vi "Host_FastOsziTest_ContAcq.vi"() -> ()   [LabVIEW 2012]
uses:
  <vilib>/FPGAPlugInAG/PXIe-7962R/niLvFpga_Open_PXIe-7962R.vi
  <vilib>/rvi/interface/common/dynamic/niFpgaDynamicAddResources.vi
  <vilib>/Utility/error.llb/Error Cluster From Error Code.vi
  <vilib>/rvi/errors/niLvFpgaAdjustHostInterfaceError.vi
  <vilib>/FPGAPlugInAG/Dynamic/niLvFpga_Close_Dynamic.vi
  <vilib>/rvi/interface/nirviOpenFPGA/nirviOpenFPGA.xnode
  FPGA Bitfiles/AnalogIntegratorFastOszi_NI5771_PXIe-7962R.lvbitx
  FPGA VIs/AnalogIntegratorFastOszi_NI5771.vi
  <vilib>/rvi/interface/nirviMethod/nirviMethod.xnode
  <vilib>/rvi/interface/nirviReadWriteControl/nirviReadWriteControl.xnode
  <vilib>/rvi/interface/nirviCloseFPGA/nirviCloseFPGA.xnode
  <vilib>/rvi/interface/Simulation/niFpgaSimulationCallBeginRW.vi
  NiFpgaLv.dll
  <vilib>/FPGAPlugInAG/Dynamic/niLvFpga_ReadFifo_Dynamic.vi
  <vilib>/rvi/errors/niLvFpgaMergeErrorWithErrorCode.vi
  <vilib>/FPGAPlugInAG/Dynamic/niLvFpga_ConfigureFifo_Dynamic.vi
panel:
  in  "Acquire continuously":bool=TRUE
  out "Configured?":bool
  out "ToHostCh1FIFO Overflow":bool
  out "InterloopFIFO Timeout":bool
  out "InterloopFIFO Overflow":bool
  in  "stop":bool
  out "Laser (Trigger In)":i16[](graph)
  in  "Samples to acquire":u32=10000
  out "IO Module\\AI Over Range":bool
  out "PMT (AI 0)":u8[](graph)
  # "Sampling at 1.5GHz => 0.66 ns sampling interval"
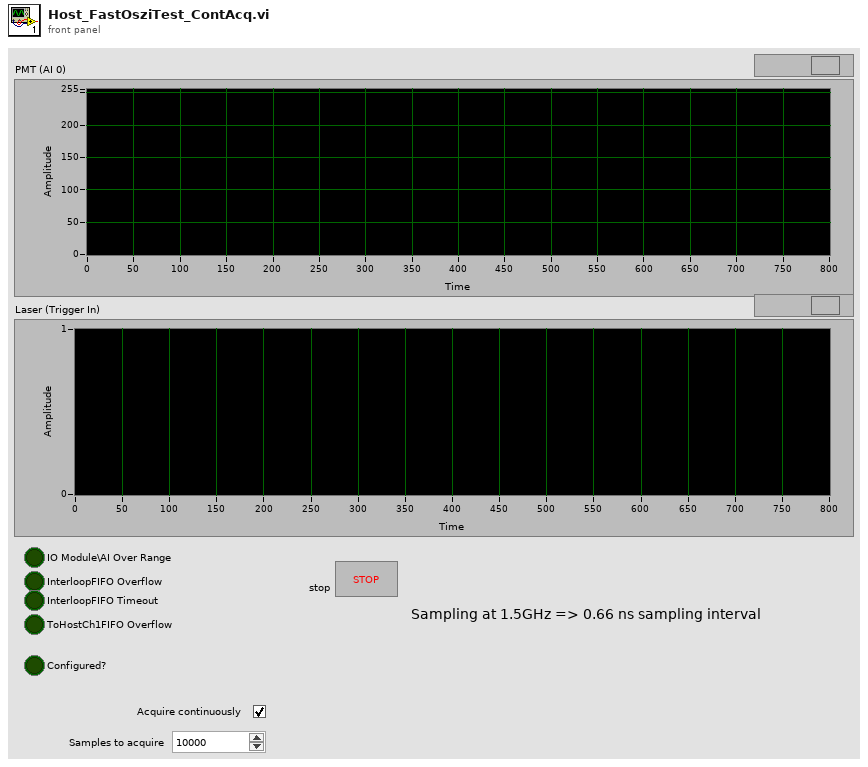
[diagram p1: front panel]
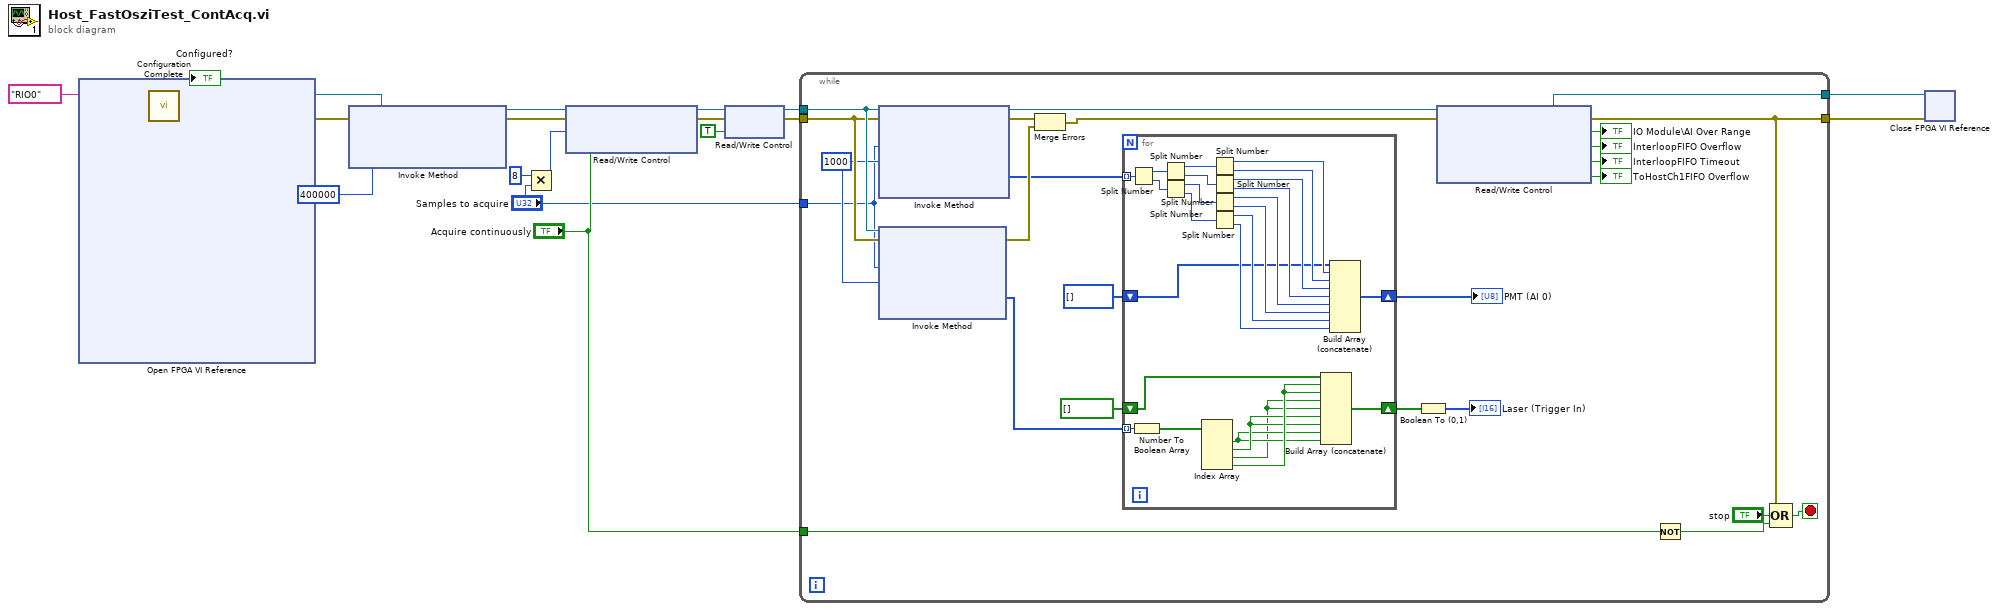
[diagram p0: block diagram]
diagram:
  n1 = xnode "Open FPGA VI Reference"("resource name"=tag "RIO0") -> ("FPGA VI Reference Out"=w15:refnum<k20>, "error out"=w19:errorcluster)  [unwired: 1 in]
  n2 = call "Configuration Complete.vi"("error in"=w19, "FPGA VI Reference In"=w15) -> ("error out"=w7:errorcluster, "Configured?"=→"Configured?":bool, "FPGA VI Reference Out"=w8:refnum<k20>)  [unwired: 7 in]
  n3 = xnode "Invoke Method"("FPGA VI Reference In"=w8, "error in"=w7, "Requested Depth"=u32 400000) -> ("FPGA VI Reference Out"=w5:refnum<k20>, "error out"=w6:errorcluster)  [unwired: 1 out]
  n4 = Multiply(x=u32 8, y="Samples to acquire") -> (x*y=w12:u32)
  n5 = xnode "Read/Write Control"("FPGA VI Reference In"=w5, "error in"=w6, "Samples to acquire"=w12, "Acquire continuously"="Acquire continuously") -> ("FPGA VI Reference Out"=w17:refnum<k20>, "error out"=w18:errorcluster)
  n6 = xnode "Read/Write Control"("FPGA VI Reference In"=w17, "error in"=w18, "Acquire"=TRUE) -> ("FPGA VI Reference Out"=w11:refnum<k20>, "error out"=w10:errorcluster)
  n7 = while {
    tunnel: [w44] -> w14
    tunnel: [w32] -> w1
    tunnel: w11 -> [w43]
    tunnel: w10 -> [w42]
    tunnel: "Acquire continuously" -> [w21]
    tunnel: "Samples to acquire" -> [w23]
    stop <- w31 stop-if-true
    w38 = 1000 ("Timeout (ms)")
    n8 = xnode "Invoke Method"("FPGA VI Reference In"=w43, "error in"=w42, "Number of Elements"=w23, "Timeout (ms)"=w38) -> ("FPGA VI Reference Out"=w45:refnum<k20>, "error out"=w41:errorcluster, "Data"=w24:u64[])  [unwired: 1 out]
    n9 = xnode "Invoke Method"("FPGA VI Reference In"=w43, "error in"=w42, "Number of Elements"=w23, "Timeout (ms)"=w38) -> ("error out"=w39:errorcluster, "Data"=w25:u8[])  [unwired: 2 out]
    n10 = Merge Errors(w41, w39) -> (w40:errorcluster)
    n11 = for {
      tunnel: w24 -> [w70] mode=indexing
      shift-right: [w55] -> w29
      shift-left: u8[] [] -> [w54]
      tunnel: w25 -> [w53] mode=indexing
      shift-right: [w48] -> w34
      shift-left: bool[] [] -> [w47]
      n12 = Split Number(x=w70) -> (hi(x)=w69:u32, lo(x)=w68:u32)
      n13 = Number To Boolean Array(number=w53) -> (Boolean array=w46:bool[])
      n14 = Split Number(x=w69) -> (hi(x)=w67:u16, lo(x)=w66:u16)
      n15 = Split Number(x=w68) -> (hi(x)=w65:u16, lo(x)=w64:u16)
      n16 = Index Array(array=w46) -> (element #1=w50:bool, element #2=w51:bool, element #3=w49:bool, element #4=w52:bool)  [unwired: 4 in]
      n17 = Split Number(x=w67) -> (hi(x)=w63:u8, lo(x)=w62:u8)
      n18 = Split Number(x=w66) -> (hi(x)=w61:u8, lo(x)=w60:u8)
      n19 = Split Number(x=w65) -> (hi(x)=w59:u8, lo(x)=w58:u8)
      n20 = Split Number(x=w64) -> (hi(x)=w57:u8, lo(x)=w56:u8)
      n21 = Build Array (concatenate)(w47, w52, w52, w49, w49, w51, w51, w50, w50) -> (w48:bool[])
      n22 = Build Array (concatenate)(w54, w63, w62, w61, w60, w59, w58, w57, w56) -> (w55:u8[])
    }
    "PMT (AI 0)" <- w29
    n23 = Boolean To (0,1)(Boolean=w34) -> (0, 1=→"Laser (Trigger In)":i16[])
    n24 = xnode "Read/Write Control"("FPGA VI Reference In"=w45, "error in"=w40) -> ("FPGA VI Reference Out"=w44:refnum<k20>, "error out"=w32:errorcluster, "IO Module\\AI Over Range"=→"IO Module\\AI Over Range":bool, "InterloopFIFO Overflow"=→"InterloopFIFO Overflow":bool, "InterloopFIFO Timeout"=→"InterloopFIFO Timeout":bool, "ToHostCh1FIFO Overflow"=→"ToHostCh1FIFO Overflow":bool)
    n25 = Not(x=w21) -> (.not. x?=w22:bool)
    n26 = Compound Arithmetic op=OR(w32, "stop", w22) -> (w31:bool)
  }
  n27 = xnode "Close FPGA VI Reference"("FPGA VI Reference In"=w14, "error in"=w1) -> ()  [unwired: 1 out]
